vi "Start Points.vi"(8 "error in":errorcluster, 11 "Sample PID Light in":refnum<class "Sample PID Light.lvclass">) -> (0 "error out":errorcluster, 3 "Sample PID Light out":refnum<class "Sample PID Light.lvclass">)   [LabVIEW 2023, in "Sample PID Light.lvclass"]
uses:
  Sample PID Light.lvclass
  Sample PID Light.lvclass/Sample PID Light.ctl
  Measure and Stimulus Subsystems/Measure and Stimulus Subsystems.lvclass
  D:/git/HAL/HAL GOOP4/Task/Task Base/Task Base.lvclass
  D:/git/HAL/HAL GOOP4/Tests/Sample Tasks/Sample PID Light/Sample PID Light.lvclass
  Task/Task Base/Task Base.lvclass
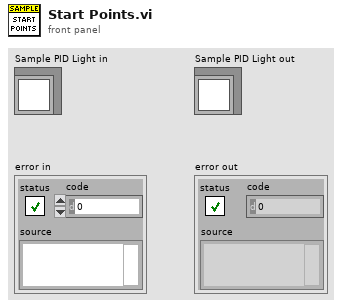
[diagram p1: front panel]
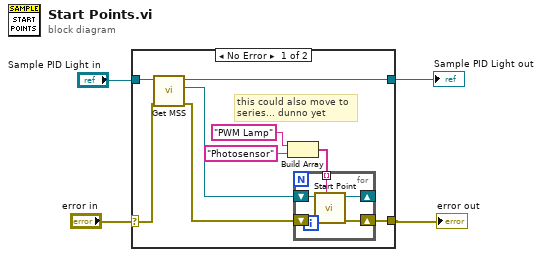
[diagram p0: block diagram]
diagram:
  n1 = case shown="No Error" "error in" {
    selector: "error in" -> [w5 w20]
    tunnel: "Sample PID Light in" -> [w13 w19]
    tunnel: [w11 w20] -> w3
    tunnel: [w6 w19] -> w1
    frame No Error {
      # "this could also move to\nseries... dunno yet"
      n2 = call "Get MSS.vi"("error in (no error)"=w5, "Task Base in"=w13) -> ("error out"=w10:errorcluster, "MSS"=w12:refnum<class "Measure and Stimulus Subsystems.lvclass">, "Task Base out"=w6:refnum<class "Sample PID Light.lvclass">)  [unwired: 7 in]
      n3 = Build Array("PWM Lamp" ("Target Ident"), "Photosensor" ("Target Identifier")) -> (w7:string[])
      n4 = for {
        shift-right: [w18] -> w11
        shift-left: w10 -> [w16]
        shift-right: [w17] -> _
        shift-left: w12 -> [w15]
        tunnel: w7 -> [w14] mode=indexing
        n5 = call "Start Point.vi"("Position Ident"=w14, "error in"=w16, "MSS in"=w15) -> ("error out"=w18:errorcluster, "MSS out"=w17:refnum<class "Measure and Stimulus Subsystems.lvclass">)  [unwired: 7 in]
      }
    }
    frame Error {
    }
  }
  "error out" <- w3
  "Sample PID Light out" <- w1
